vi "PrepLineObjectArray_write_and_unlock.vi"(8 "error in (no error)":errorcluster, 11 "PrepLineObjArray":refnum<class "PrepLineObject.lvclass">[](array[class])) -> (0 "error out":errorcluster)   [LabVIEW 2013]
doc: "the VI unlocks the PreplineObjectArray and writes the array data into the global variable"
uses:
  Classes/PrepLineObject/PrepLineObject.lvclass
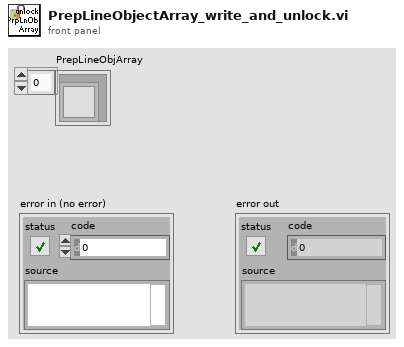
[diagram p1: front panel]
types:
  T1 = typedef "Semaphore RefNum" = refnum<k1>
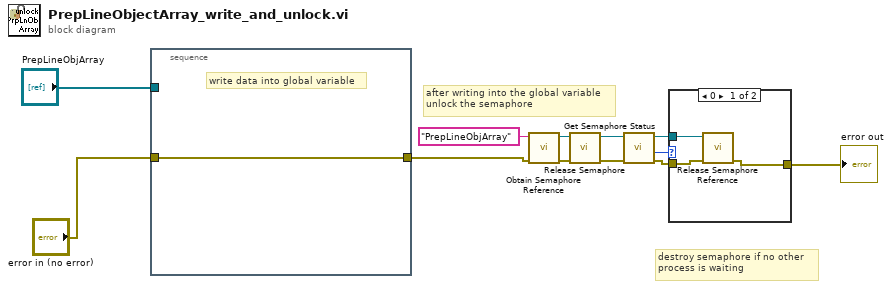
[diagram p0: block diagram]
diagram:
  # "destroy semaphore if no other\nprocess is waiting"
  # "after writing into the global variable\nunlock the semaphore"
  n1 = stacked-sequence {
    tunnel: "error in (no error)" -> [w13]
    tunnel: "PrepLineObjArray" -> [_]
    tunnel: [w13] -> w7
    frame #0 {
      # "write data into global variable"
    }
  }
  n2 = call <vilib>:"Obtain Semaphore Reference.vi"("error in (no error)"=w7, "name (unnamed)"="PrepLineObjArray") -> ("error out"=w10:errorcluster, "semaphore"=w11:T1)  [unwired: 3 in, 1 out]
  n3 = call <vilib>:"Release Semaphore.vi"("error in (no error)"=w10, "semaphore"=w11) -> ("error out"=w6:errorcluster, "semaphore out"=w5:T1)  [unwired: 4 in]
  n4 = call <vilib>:"Get Semaphore Status.vi"("error in (no error)"=w6, "semaphore"=w5) -> ("error out"=w2:errorcluster, "# waiting"=w4:i32, "semaphore out"=w3:T1)  [unwired: 4 in, 3 out]
  n5 = case shown="0" w4 {
    tunnel: w3 -> [w16 _]
    tunnel: w2 -> [w15 w17]
    tunnel: [w14 w17] -> w1
    frame 0 {
      n6 = call <vilib>:"Release Semaphore Reference.vi"("error in (no error)"=w15, "semaphore"=w16) -> ("error out"=w14:errorcluster)  [unwired: 8 in, 1 out]
    }
    frame 1, Default {
    }
  }
  "error out" <- w1
